vi "Event Capture Sim Test.vi"() -> ()   [LabVIEW 2015]
uses:
  IP Source/ECU Event/Timing/Measure Output.ctl
  IP Source/APU/Shared Settings.ctl
  IP Source/APU/Input.ctl
  Simulation FPGA/Event Gen Config.ctl
  IP Source/ECU Event/Timing/Measure Settings.ctl
  <vilib>/rvi/interface/RandomDataEmulation/nirviRandomDataOpen.vi
  <vilib>/rvi/interface/common/niFpgaCacheSessionInfoDynamic.vi
  <vilib>/Utility/error.llb/Error Cluster From Error Code.vi
  <vilib>/rvi/errors/niLvFpgaAdjustHostInterfaceError.vi
  <vilib>/FPGAPlugInAG/Dynamic/niLvFpga_Run_Dynamic.vi
  <vilib>/FPGAPlugInAG/Dynamic/niLvFpga_Close_Dynamic.vi
  <vilib>/rvi/interface/nirviOpenFPGA/nirviOpenFPGA.xnode
  Simulation FPGA/APU + Event Timing 40MHz.vi
  Simulation FPGA/APU + Event Timing.vi
  <vilib>/rvi/interface/nirviReadWriteControl/nirviReadWriteControl.xnode
  <vilib>/rvi/interface/nirviMethod/nirviMethod.xnode
  <vilib>/rvi/interface/nirviCloseFPGA/nirviCloseFPGA.xnode
  IP Source/APU/APU.lvlib
  <vilib>/rvi/interface/Simulation/niFpgaSimulationCallBeginRW.vi
  IP Source/ECU Event/Timing/ECU Event Timing.lvlib
  NiFpgaLv.dll
panel:
  in  "crank start (U16s)":u16
  in  "40MHz Events":bool
  in  "time before stuck active (ms)":dbl=1.0 min=0.0 max=209.7152 step=0.0016
  out "status.spark 1":T1
  in  "Reset":bool
  out "Speed":dbl(graph)
  out "capture.Spark 1 Shot 2":T2
  out "capture.Spark 1 Shot 1":T2
  in  "Settings.Spark 1":T3={"Max"=100.0, "Min"=10.0, "active high"=TRUE}
  in  "Other Pulse Config":T4={"Gen Event"=FALSE, "Gen Event Start"=50.0, "Gen Event Duration (ms)"=0.02}
  in  "Pulse Config":T4={"Gen Event"=FALSE, "Gen Event Start"=2.0, "Gen Event Duration (ms)"=0.015}
  out "Cycle Angle":dbl(graph)
  in  "RPM":dbl=73242.2 format="%#_15g"
  in  "stop":bool
  # "Simulated ECU settings"
  # "Engine Sim Settings"
  # "Run Time Data"
  # "1ms duration is 440 degrees at max RPM. 1.64ms is 720 degrees.\n0.227ms is 100 degrees"
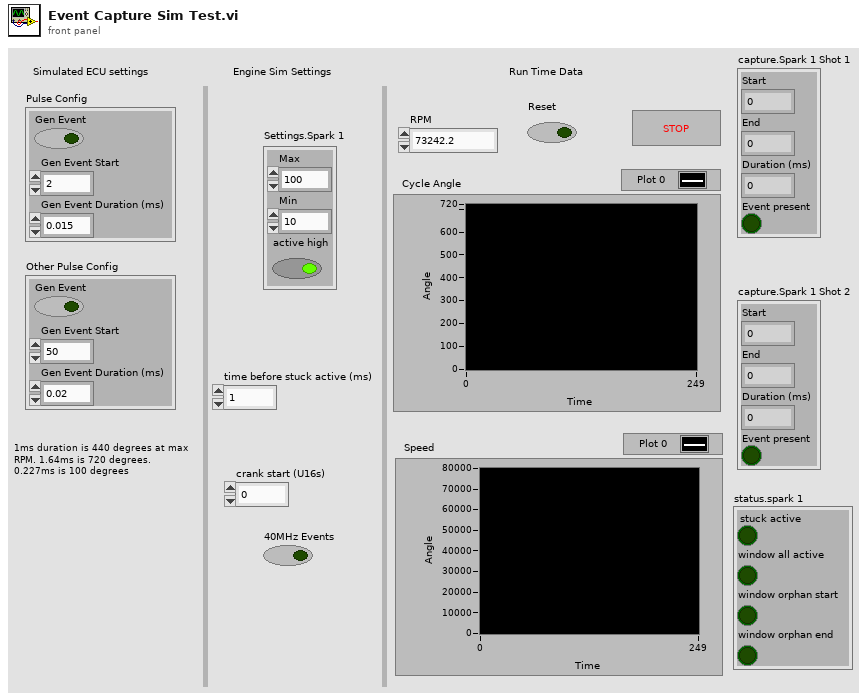
[diagram p1: front panel]
types:
  T1 = typedef "Engine Simulation Toolkit.lvlib/ECU Event Timing.lvlib/Measure Output.ctl" = cluster{"stuck active":bool, "window all active":bool, "window orphan start":bool, "window orphan end":bool}
  T2 = cluster{"Start":dbl, "End":dbl, "Duration (ms)":dbl, "Event present":bool}
  T3 = cluster{"Max":dbl, "Min":dbl, "active high":bool}
  T4 = cluster{"Gen Event":bool, "Gen Event Start":dbl, "Gen Event Duration (ms)":dbl}
  T5 = typedef "Engine Simulation Toolkit.lvlib/APU.lvlib/Shared Settings.ctl" = cluster{"start":fxp<+,17,17>, "stuck limit":fxp<+,18,18>}
  T6 = typedef "Engine Simulation Toolkit.lvlib/ECU Event Timing.lvlib/Measure Settings.ctl" = cluster{"max":u16, "min":u16, "active high":bool, "wrap":bool}
  T7 = typedef "Engine Simulation Toolkit.lvlib/APU.lvlib/Input.ctl" = cluster{"desired speed":fxp<+/-,23,2>, "reset":bool}
  T8 = typedef "Event Gen Config.ctl" = cluster{"Gen Event":bool, "Gen Event Start":u16, "Gen Event Duration (tics)":u32}
  T9 = cluster{"stuck active":bool, "window all active":bool, "window orphan start":bool, "window orphan end":bool}
  T10 = cluster{"Start":u16, "End":u16, "Duration (tics)":fxp<+,18,18>, "Event present":bool}
  T11 = cluster{"crank":u16, "cycle":u16, "actual speed":fxp<+/-,23,2>}
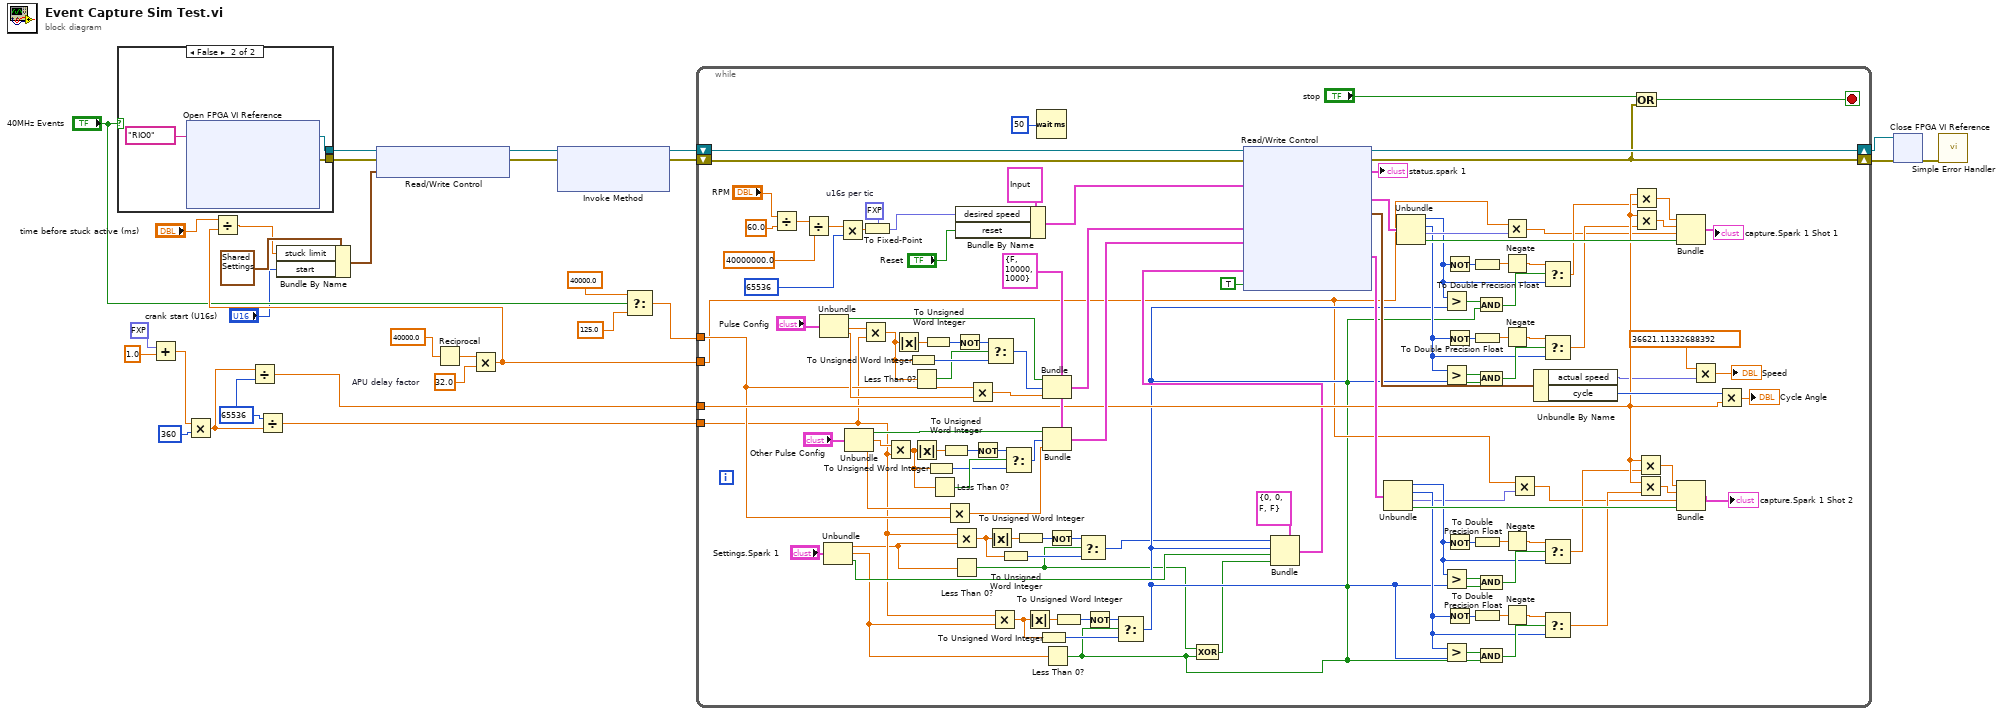
[diagram p0: block diagram]
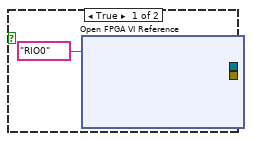
[diagram p2: hidden frame]
diagram:
  w18 = u32 65536 ("y")
  w23 = 32.0  # APU delay factor
  n1 = case shown="False" "40MHz Events" {
    tunnel: [w33 w36] -> w27
    tunnel: [w31 w34] -> w25
    frame True {
      n2 = xnode "Open FPGA VI Reference"("resource name"=tag "RIO0") -> ("FPGA VI Reference Out"=w31:refnum<k20>, "error out"=w33:errorcluster)  [unwired: 1 in]
    }
    frame False {
      n3 = xnode "Open FPGA VI Reference"("resource name"=tag "RIO0") -> ("FPGA VI Reference Out"=w34:refnum<k20>, "error out"=w36:errorcluster)  [unwired: 1 in]
    }
  }
  n4 = Add(x=fxp<+,2,2> 1.0 ("extra cranks for a cycle"), y=1.0) -> (x+y=w19:dbl)
  n5 = Multiply(x=w19, y=u16 360) -> (x*y=w16:dbl)
  n6 = Divide(x=w16, y=w18) -> (x/y=w17:dbl)
  n7 = Divide(x=w18, y=w16) -> (x/y=w15:dbl)
  n8 = Reciprocal(x=40000.0) -> (1/x=w24:dbl)
  n9 = Multiply(x=w24, y=w23) -> (x*y=w13:dbl)
  n10 = Divide(x="time before stuck active (ms)", y=w13) -> (x/y=w10:dbl)
  n11 = Bundle By Name(cluster=T5 {"start"=0.0, "stuck limit"=0.0} ("APU Shared Settings"), "stuck limit"=w10, "start"="crank start (U16s)") -> (w11:T5)
  n12 = xnode "Read/Write Control"("FPGA VI Reference In"=w25, "error in"=w27, "shared settings.my apu"=w11) -> ("FPGA VI Reference Out"=w8:refnum<k20>, "error out"=w26:errorcluster)
  n13 = xnode "Invoke Method"("FPGA VI Reference In"=w8, "error in"=w26) -> ("FPGA VI Reference Out"=w7:refnum<k20>, "error out"=w9:errorcluster)  [unwired: 1 in]
  n14 = Select(t=40000.0 ("x"), s="40MHz Events", f=125.0 ("x")) -> (s? t:f=w2:dbl)
  n15 = while {
    shift-right: [w152] -> w30
    shift-left: w9 -> [w157]
    shift-right: [w155] -> w29
    shift-left: w7 -> [w156]
    tunnel: w17 -> [w116]
    tunnel: w15 -> [w42]
    tunnel: w2 -> [w62]
    tunnel: w13 -> [w49]
    stop <- w153 stop-if-true
    w135 = T8 {"Gen Event"=FALSE, "Gen Event Start"=10000, "Gen Event Duration (tics)"=1000} ("Pulse Config")
    w142 = fxp<+/-,23,2> 0.0  # u16s per tic
    n16 = Divide(x="RPM", y=60.0) -> (x/y=w147:dbl)
    n17 = Divide(x=w147, y=40000000.0) -> (x/y=w143:dbl)
    n18 = Unbundle("Pulse Config") -> ("Gen Event"=w132:bool, "Gen Event Start"=w133:dbl, "Gen Event Duration (ms)"=w65:dbl)
    n19 = Unbundle("Settings.Spark 1") -> ("Max"=w41:dbl, "Min"=w50:dbl, "active high"=w128:bool)
    n20 = Multiply(x=w143, y=u32 65536 ("n")) -> (x*y=w141:dbl)
    n21 = Unbundle("Other Pulse Config") -> ("Gen Event"=w134:bool, "Gen Event Start"=w131:dbl, "Gen Event Duration (ms)"=w63:dbl)
    n22 = Multiply(x=w133, y=w42) -> (x*y=w91:dbl)
    n23 = To Fixed-Point(fixed-point type=w142, number=w141) -> (fixed-point=w140:fxp<+/-,23,2>)
    n24 = Multiply(x=w131, y=w42) -> (x*y=w84:dbl)
    n25 = Absolute Value(x=w91) -> (abs(x)=w95:dbl)
    n26 = To Unsigned Word Integer(number=w91) -> (unsigned 16bit integer=w93:u16)
    n27 = Less Than 0?(x=w91) -> (x < 0?=w92:bool)
    n28 = Absolute Value(x=w84) -> (abs(x)=w86:dbl)
    n29 = To Unsigned Word Integer(number=w95) -> (unsigned 16bit integer=w96:u16)
    n30 = To Unsigned Word Integer(number=w84) -> (unsigned 16bit integer=w88:u16)
    n31 = Less Than 0?(x=w84) -> (x < 0?=w89:bool)
    n32 = To Unsigned Word Integer(number=w86) -> (unsigned 16bit integer=w85:u16)
    n33 = Multiply(x=w63, y=w62) -> (x*y=w61:dbl)
    n34 = Multiply(x=w42, y=w41) -> (x*y=w44:dbl)
    n35 = Less Than 0?(x=w41) -> (x < 0?=w38:bool)
    n36 = Not(x=w96) -> (.not. x?=w94:u16)
    n37 = Bundle By Name(cluster=T7 {"desired speed"=0.0, "reset"=FALSE} ("my apu"), "desired speed"=w140, "reset"="Reset") -> (w149:T7)
    n38 = Multiply(x=w62, y=w65) -> (x*y=w64:dbl)
    n39 = Not(x=w85) -> (.not. x?=w87:u16)
    n40 = Select(t=w94, s=w92, f=w93) -> (s? t:f=w90:u16)
    n41 = Absolute Value(x=w44) -> (abs(x)=w45:dbl)
    n42 = Multiply(x=w42, y=w50) -> (x*y=w112:dbl)
    n43 = To Unsigned Word Integer(number=w44) -> (unsigned 16bit integer=w47:u16)
    n44 = Select(t=w87, s=w89, f=w88) -> (s? t:f=w83:u16)
    n45 = To Unsigned Word Integer(number=w45) -> (unsigned 16bit integer=w43:u16)
    n46 = Absolute Value(x=w112) -> (abs(x)=w111:dbl)
    n47 = Wait (ms)(milliseconds to wait=u32 50) -> ()  [unwired: 1 out]
    n48 = To Unsigned Word Integer(number=w112) -> (unsigned 16bit integer=w109:u16)
    n49 = Bundle(cluster=w135, "Gen Event"=w132, "Gen Event Start"=w90, "Gen Event Duration (tics)"=w64) -> (w126:T8)
    n50 = Bundle(cluster=w135, "Gen Event"=w134, "Gen Event Start"=w83, "Gen Event Duration (tics)"=w61) -> (w127:T8)
    n51 = Less Than 0?(x=w50) -> (x < 0?=w37:bool)
    n52 = Not(x=w43) -> (.not. x?=w46:u16)
    n53 = To Unsigned Word Integer(number=w111) -> (unsigned 16bit integer=w113:u16)
    n54 = Select(t=w46, s=w38, f=w47) -> (s? t:f=w40:u16)
    n55 = Not(x=w113) -> (.not. x?=w110:u16)
    n56 = Select(t=w110, s=w37, f=w109) -> (s? t:f=w66:u16)
    n57 = Exclusive Or(1:w37, 2:w38) -> (0:w39:bool)
    n58 = Bundle(cluster=T6 {"max"=0, "min"=0, "active high"=FALSE, "wrap"=FALSE} ("Settings.Spark 1"), "max"=w40, "min"=w66, "active high"=w128, "wrap"=w39) -> (w115:T6)
    n59 = xnode "Read/Write Control"("FPGA VI Reference In"=w156, "error in"=w157, "input.my apu"=w149, "Pulse Config"=w126, "Other Pulse Config"=w127, "settings.spark 1"=w115, "go.my apu"=TRUE) -> ("FPGA VI Reference Out"=w155:refnum<k20>, "error out"=w152:errorcluster, "status.spark 1"=→"status.spark 1":T9, "capture.spark 1.Shot 1"=w117:T10, "output.my apu"=w148:T11, "capture.spark 1.Shot 2"=w125:T10)
    n60 = Unbundle(w125) -> ("Start"=w70:u16, "End"=w69:u16, "Duration (tics)"=w60:fxp<+,18,18>, "Event present"=w122:bool)
    n61 = Unbundle(w117) -> ("Start"=w97:u16, "End"=w100:u16, "Duration (tics)"=w120:fxp<+,18,18>, "Event present"=w121:bool)
    n62 = Greater?(x=w97, y=w66) -> (0:w82:bool)
    n63 = Greater?(x=w100, y=w66) -> (0:w81:bool)
    n64 = Greater?(x=w70, y=w66) -> (0:w79:bool)
    n65 = Greater?(x=w69, y=w66) -> (0:w80:bool)
    n66 = Not(x=w97) -> (.not. x?=w101:u16)
    n67 = Not(x=w100) -> (.not. x?=w108:u16)
    n68 = Not(x=w70) -> (.not. x?=w78:u16)
    n69 = Not(x=w69) -> (.not. x?=w71:u16)
    n70 = To Double Precision Float(number=w101) -> (double precision float=w102:dbl)
    n71 = To Double Precision Float(number=w108) -> (double precision float=w107:dbl)
    n72 = To Double Precision Float(number=w78) -> (double precision float=w77:dbl)
    n73 = To Double Precision Float(number=w71) -> (double precision float=w72:dbl)
    n74 = And(x=w82, y=w37) -> (x .and. y?=w104:bool)
    n75 = And(x=w81, y=w37) -> (x .and. y?=w105:bool)
    n76 = And(x=w79, y=w37) -> (x .and. y?=w75:bool)
    n77 = And(x=w80, y=w37) -> (x .and. y?=w74:bool)
    n78 = Multiply(x=w49, y=w120) -> (x*y=w58:dbl)
    n79 = Negate(x=w102) -> (-x=w103:dbl)
    n80 = Negate(x=w107) -> (-x=w106:dbl)
    n81 = Negate(x=w77) -> (-x=w76:dbl)
    n82 = Negate(x=w72) -> (-x=w73:dbl)
    n83 = Multiply(x=w49, y=w60) -> (x*y=w59:dbl)
    n84 = Unbundle By Name(w148) -> ("actual speed"=w54:fxp<+/-,23,2>, "cycle"=w139:u16)
    n85 = Select(t=w103, s=w104, f=w97) -> (s? t:f=w98:dbl)
    n86 = Select(t=w106, s=w105, f=w100) -> (s? t:f=w99:dbl)
    n87 = Select(t=w76, s=w75, f=w70) -> (s? t:f=w68:dbl)
    n88 = Select(t=w73, s=w74, f=w69) -> (s? t:f=w67:dbl)
    n89 = Or(x="stop", y=w152) -> (x .or. y?=w153:bool)
    n90 = Multiply(x=w116, y=w98) -> (x*y=w118:dbl)
    n91 = Multiply(x=w116, y=w99) -> (x*y=w119:dbl)
    n92 = Multiply(x=w116, y=w68) -> (x*y=w124:dbl)
    n93 = Multiply(x=w116, y=w67) -> (x*y=w123:dbl)
    n94 = Bundle(w118, w119, w58, "Event present"=w121) -> (→"capture.Spark 1 Shot 1":cluster{dbl, dbl, dbl, "Event present":bool})  [unwired: 1 in]
    n95 = Bundle(w124, w123, w59, "Event present"=w122) -> (→"capture.Spark 1 Shot 2":cluster{dbl, dbl, dbl, "Event present":bool})  [unwired: 1 in]
    n96 = Multiply(x=36621.11332688392 ("y"), y=w54) -> (x*y=→"Speed":dbl)
    n97 = Multiply(x=w139, y=w116) -> (x*y=→"Cycle Angle":dbl)
  }
  n98 = xnode "Close FPGA VI Reference"("FPGA VI Reference In"=w29, "error in"=w30) -> ("error out"=w28:errorcluster)
  n99 = call <vilib>:"Simple Error Handler.vi"("error in (no error)"=w28) -> ()  [unwired: 4 in, 5 out]
